vi "Initialise.vi"(8 "VIA":refnum<vi>, 9 "RAM":refnum<vi>, 10 "EEPROM":refnum<vi>, 11 "ROM":path) -> (0 "VIA Viewer":refnum<class "Hex Viewer.lvclass">, 1 "RAM Viewer":refnum<class "Hex Viewer.lvclass">, 2 "EEPROM Viewer":refnum<class "Hex Viewer.lvclass">, 3 "IO out":refnum<class "IO.lvclass">)   [LabVIEW 2021]
uses:
  IO/IO.lvclass
  Hex Viewer/Hex Viewer.lvclass
  Memory/Memory.lvclass/Memory.ctl
  IO/IO.lvclass/IO.ctl
  Memory Map/Memory Map.lvclass
  Memory/Memory.lvclass
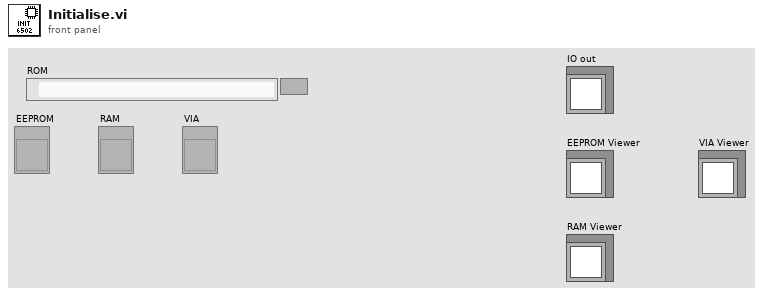
[diagram p1: front panel]
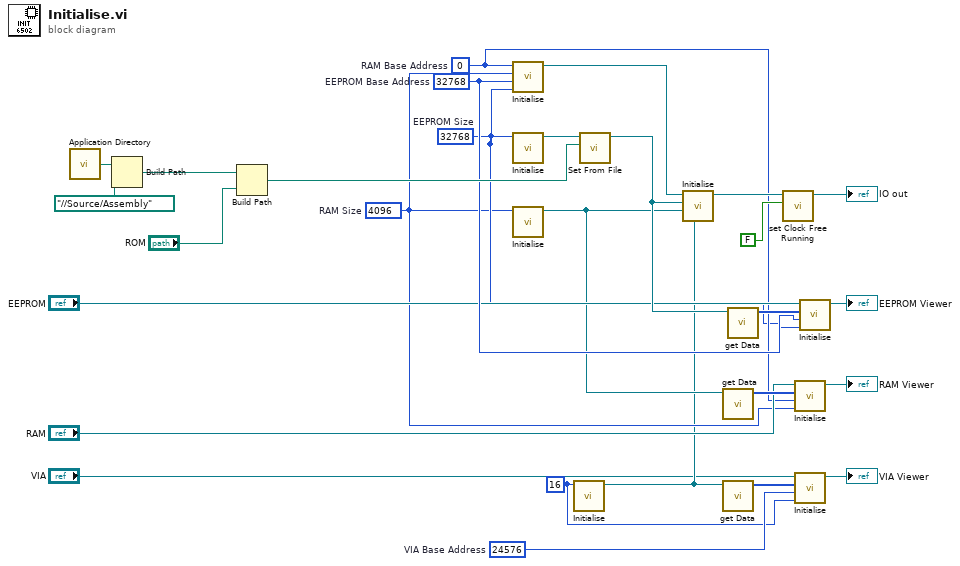
[diagram p0: block diagram]
diagram:
  w4 = u16 24576  # VIA Base Address
  w3 = u16 16 ("Size")
  w16 = u16 32768  # EEPROM Base Address
  w9 = u16 0  # RAM Base Address
  w7 = u16 4096  # RAM Size
  w8 = u16 32768  # EEPROM Size
  n1 = call <vilib>:"Application Directory.vi"() -> ("Application Directory"=w20:path)
  n2 = Build Path(base path=w20, name or relative path=path "../../Source/Assembly" ("ROM")) -> (appended path=w22:path)
  n3 = Build Path(base path=w22, name or relative path="ROM") -> (appended path=w24:path)
  n4 = call "Initialise.vi"("EEPROM Size"=w8, "EEPROM Base Address"=w16, "RAM Size"=w7, "RAM Base Address"=w9) -> ("Memory Map out"=w28:refnum<class "Memory Map.lvclass">)  [unwired: 7 in]
  n5 = call "Initialise.vi"("Size"=w8) -> ("Memory out"=w19:refnum<class "Memory.lvclass">)  [unwired: 10 in]
  n6 = call "Initialise.vi"("Size"=w7) -> ("Memory out"=w11:refnum<class "Memory.lvclass">)  [unwired: 10 in]
  n7 = call "Initialise.vi"("Size"=w3) -> ("Memory out"=w2:refnum<class "Memory.lvclass">)  [unwired: 10 in]
  n8 = call "Set From File.vi"("Memory binary"=w24, "Memory in"=w19) -> ("Memory out"=w17:refnum<class "Memory.lvclass">)  [unwired: 8 in, 1 out]
  n9 = call "Initialise.vi"("VIA"=w2, "RAM"=w11, "EEPROM"=w17, "Memory Map"=w28) -> ("Clock Generator"=w25:refnum<class "IO.lvclass">)  [unwired: 6 in, 1 out]
  n10 = call "get Data.vi"("Memory in"=w11) -> ("Data"=w12:u8[])  [unwired: 10 in]
  n11 = call "get Data.vi"("Memory in"=w2) -> ("Data"=w6:u8[])  [unwired: 10 in]
  n12 = call "get Data.vi"("Memory in"=w17) -> ("Data"=w18:u8[])  [unwired: 10 in]
  n13 = call "set Clock Free Running.vi"("Free Running"=FALSE, "Clock Generator in"=w25) -> ("Clock Generator out"=→"IO out":refnum<class "IO.lvclass">)  [unwired: 9 in]
  n14 = call "Initialise.vi"("Size"=w7, "Offset"=w9, "Data"=w12, "Table"="RAM") -> ("Hex Viewer"=→"RAM Viewer":refnum<class "Hex Viewer.lvclass">)  [unwired: 7 in]
  n15 = call "Initialise.vi"("Size"=w3, "Offset"=w4, "Data"=w6, "Table"="VIA") -> ("Hex Viewer"=→"VIA Viewer":refnum<class "Hex Viewer.lvclass">)  [unwired: 7 in]
  n16 = call "Initialise.vi"("Size"=w8, "Offset"=w16, "Data"=w18, "Table"="EEPROM") -> ("Hex Viewer"=→"EEPROM Viewer":refnum<class "Hex Viewer.lvclass">)  [unwired: 7 in]
